vi "MapChannels.vi"(8 "error in (no error)":errorcluster caption="错误输入（无错误）", 11 "TPlot 输入":refnum<class "TPlot.lvclass">) -> (0 "error out":errorcluster caption="错误输出", 3 "TPlot 输出":refnum<class "TPlot.lvclass">)   [LabVIEW 2018, in "DataDisplay.lvlib" / "TPlot.lvclass"]
uses:
  TPlot.lvclass
  TPlot.lvclass/TPlot.ctl
  DataDisplay.lvlib
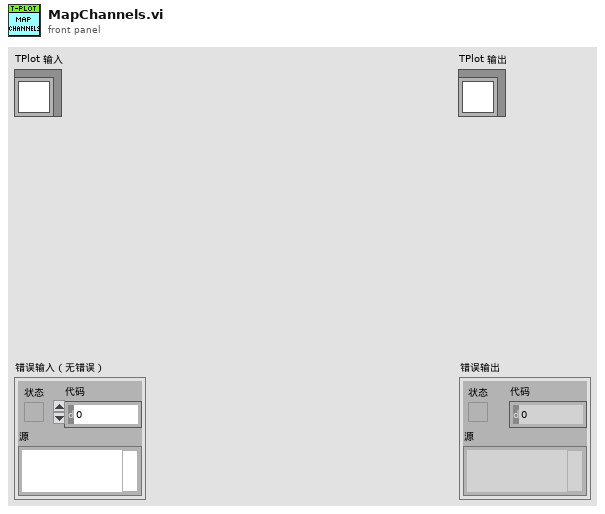
[diagram p1: front panel]
types:
  T1 = typedef "DataDisplay.lvlib/DD_CommandQ.ctl" = refnum<queue>
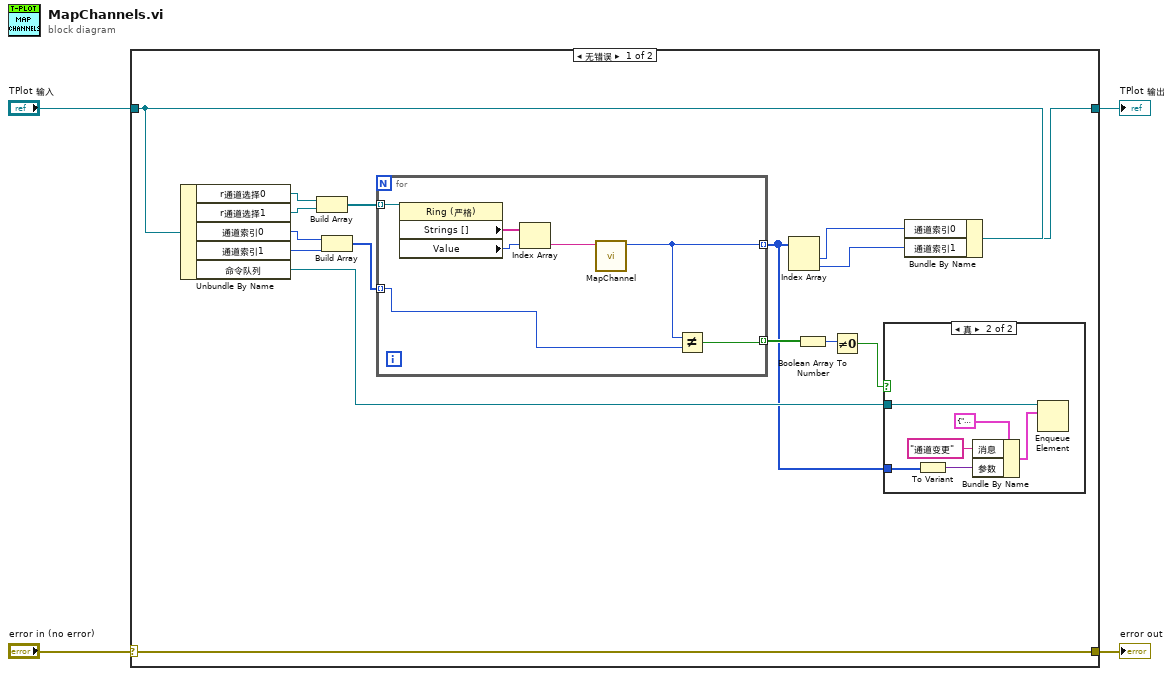
[diagram p0: block diagram]
diagram:
  n1 = case shown="无错误" "error in (no error)" {
    selector: "error in (no error)" -> [w20 w35]
    tunnel: [w20 w35] -> w3
    tunnel: [w8 w34] -> w1
    tunnel: "TPlot 输入" -> [w19 w34]
    frame No Error {
      n2 = Unbundle By Name(w19) -> ("r通道选择0"=w18:refnum<vi>, "r通道选择1"=w17:refnum<vi>, "通道索引0"=w15:i32, "通道索引1"=w14:i32, "命令队列"=w12:T1)
      n3 = Build Array(w18, w17) -> (w16:refnum<vi>[])
      n4 = Build Array(w15, w14) -> (w13:i32[])
      n5 = for {
        tunnel: w16 -> [w33] mode=indexing
        tunnel: w13 -> [w28] mode=indexing
        tunnel: [w29] -> w11 mode=indexing
        tunnel: [w27] -> w5 mode=indexing
        n6 = property class="Ring (严格)"(reference=w33) -> ("Strings []"=w32:string[], "Value"=w31:u16)  [unwired: 1 in, 2 out]
        n7 = Index Array(array=w32, index=w31) -> (element=w30:string)
        n8 = call "MapChannel.vi"("通道名称"=w30) -> ("索引"=w27:i32)  [unwired: 9 in, 1 out]
        n9 = Not Equal?(x=w27, y=w28) -> (x != y?=w29:bool)
      }
      n10 = Index Array(array=w5) -> (element #1=w7:i32, element #2=w6:i32)  [unwired: 2 in]
      n11 = Boolean Array To Number(Boolean array=w11) -> (number=w10:u32)
      n12 = Not Equal To 0?(x=w10) -> (x != 0?=w9:bool)
      n13 = case shown="真" w9 {
        tunnel: w12 -> [_ w26]
        tunnel: w5 -> [_ w22]
        frame False {
        }
        frame True {
          n14 = To Variant(anything=w22) -> (Variant=w23:variant)
          n15 = Bundle By Name(cluster=cluster{"消息":string, "参数":variant} {"消息"="", "参数"=variant} ("元素"), "消息"="通道变更", "参数"=w23) -> (w21:cluster{"消息":string, "参数":variant})
          n16 = Enqueue Element(queue=w26, element=w21) -> ()  [unwired: 2 in, 3 out]
        }
      }
      n17 = Bundle By Name(cluster=w19, "通道索引0"=w7, "通道索引1"=w6) -> (w8:refnum<class "TPlot.lvclass">)
    }
    frame Error {
    }
  }
  "error out" <- w3
  "TPlot 输出" <- w1
